vi "wait_for_connection_process.vi"(9 "Notifier":refnum<notifier>, 10 "Queue":refnum<queue>, 11 "Connection":refnum<class "Connection.lvclass">) -> ()   [LabVIEW 2013, in "Connection_GOSPL.lvlib" / "Connection.Collection.lvclass"]
uses:
  Connection.Collection.lvclass
  Connection/Connection.lvclass
  incoming connection.ctl
  map.ctl
  Connection/Connection.lvclass/Connection.ctl
panel:
  out "error out":errorcluster
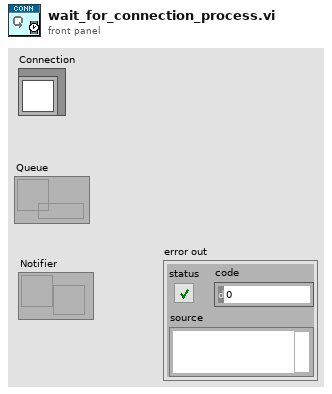
[diagram p1: front panel]
types:
  T1 = typedef "Connection_GOSPL.lvlib/Connection.Collection.lvclass/incoming connection.ctl" = cluster{"Connection":refnum<class "Connection.lvclass">, "error":errorcluster}
  T2 = typedef "Connection_GOSPL.lvlib/Connection.Collection.lvclass/map.ctl" = cluster{"Connection":refnum<class "Connection.lvclass">, "Queue":refnum<queue>}
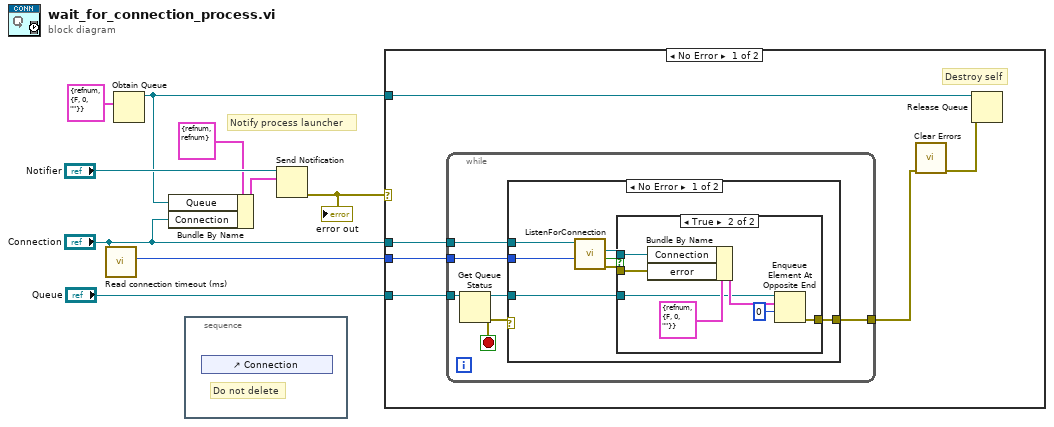
[diagram p0: block diagram]
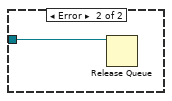
[diagram p4: hidden frame]
diagram:
  # "Notify process launcher"
  n1 = call "Read connection timeout (ms).vi"("Connection in"="Connection") -> ("connection timeout (ms)"=w1:i32)  [unwired: 8 in, 2 out]
  n2 = Obtain Queue(element data type=T1 {"Connection"=refnum, "error"={"status"=FALSE, "code"=0, "source"=""}}) -> (queue out=w4:refnum<queue>)  [unwired: 4 in, 2 out]
  n3 = Bundle By Name(cluster=T2 {"Connection"=refnum, "Queue"=refnum} ("notification"), "Queue"=w4, "Connection"="Connection") -> (w7:T2)
  n4 = stacked-sequence {
    frame #0 {
      # "Do not delete"
      n5 = control-ref of="Connection"() -> ()  [unwired: 1 out]
    }
  }
  n6 = Send Notification(notification=w7, notifier="Notifier") -> (error out=w3:errorcluster)  [unwired: 1 in, 1 out]
  "error out" <- w3
  n7 = case shown="No Error" w3 {
    tunnel: w1 -> [w15 _]
    tunnel: "Queue" -> [w14 _]
    tunnel: "Connection" -> [w12 _]
    tunnel: w4 -> [w13 w37]
    frame No Error {
      # "Destroy self"
      n8 = while {
        tunnel: w15 -> [w21]
        tunnel: w14 -> [w18]
        tunnel: w12 -> [w20]
        tunnel: [w19] -> w10
        stop <- w16 stop-if-true
        n9 = Get Queue Status(queue=w18) -> (queue out=w17:refnum<queue>, error out=w16:errorcluster)  [unwired: 2 in, 6 out]
        n10 = case shown="No Error" w16 {
          tunnel: w21 -> [w22 _]
          tunnel: w20 -> [w26 _]
          tunnel: [w25 _] -> w19
          tunnel: w17 -> [w24 _]
          frame No Error {
            n11 = call "ListenForConnection.vi"("timeout (2000 ms)"=w22, "Listener"=w26) -> ("error out"=w28:errorcluster, "New connection"=w23:bool, "Connection"=w27:refnum<class "Connection.lvclass">)  [unwired: 6 in, 1 out]
            n12 = case shown="True" w23 {
              tunnel: w28 -> [w29 w36]
              tunnel: w27 -> [_ w32]
              tunnel: [w29 w31] -> w25
              tunnel: w24 -> [_ w30]
              frame False {
              }
              frame True {
                n13 = Bundle By Name(cluster=T1 {"Connection"=refnum, "error"={"status"=FALSE, "code"=0, "source"=""}} ("Connection_GOSPL.lvlib:Connection.Collection.lvclass:incoming connection"), "Connection"=w32, "error"=w36) -> (w34:T1)
                n14 = Enqueue Element At Opposite End(queue=w30, element=w34, timeout in ms (-1)=0) -> (error out=w31:errorcluster)  [unwired: 1 in, 2 out]
              }
            }
          }
          frame Error {
          }
        }
      }
      n15 = call <vilib>:"Clear Errors.vi"("error in (no error)"=w10) -> ("error out"=w11:errorcluster)  [unwired: 6 in]
      n16 = Release Queue(queue=w13, error in (no error)=w11) -> ()  [unwired: 1 in, 3 out]
    }
    frame Error {
      n17 = Release Queue(queue=w37) -> ()  [unwired: 2 in, 3 out]
    }
  }
